vi "FluxMeasure.vi"(4 "On/Off":bool, 5 "error in (no error)":errorcluster, 6 "Gray Image":T1) -> (0 "error out":errorcluster, 1 "实时通量":cluster{"粒子数量":dbl, "粒子数量":dbl, dbl}, 2 "粒子分布":cluster{dbl[], i32[]}, 3 "粒子数量":dbl)   [LabVIEW 2012]
uses:
  <vilib>/vision/Image Controls.llb/IMAQ Image.ctl
  <vilib>/vision/NI_Vision_Development_Module.lvlib
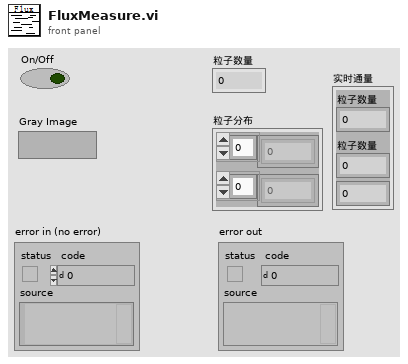
[diagram p1: front panel]
types:
  T1 = typedef "IMAQ Image.ctl" = refnum<image>
  T2 = typedef "Particle Parameters" = i32
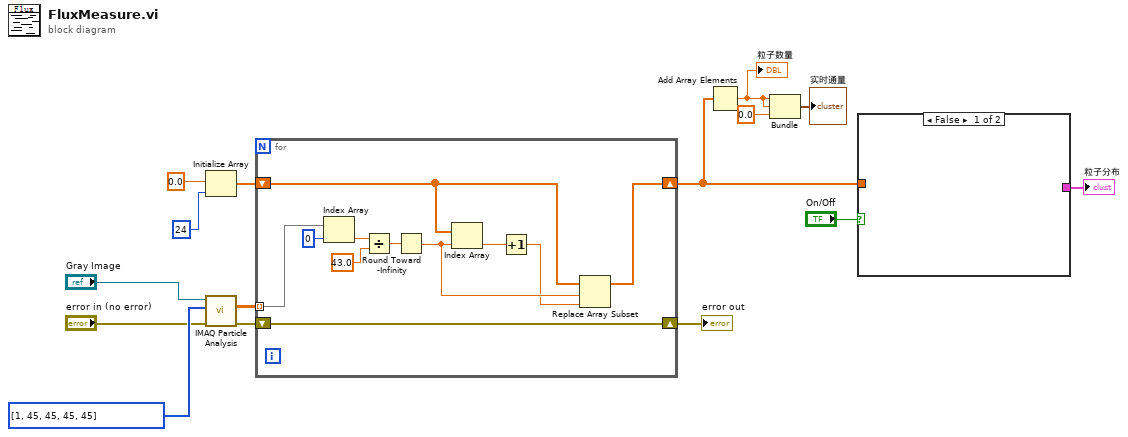
[diagram p0: block diagram]
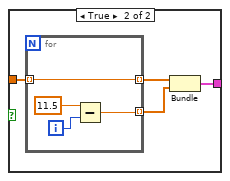
[diagram p2: hidden frame]
diagram:
  w15 = T2[] [1, 45, 45, 45, 45] items=["Center of Mass X", "Center of Mass Y", "First Pixel X", "First Pixel Y", "Bounding Rect Left", "Bounding Rect Top", "Bounding Rect Right", "Bounding Rect Bottom", "Max Feret Diameter Start X", "Max Feret Diameter Start Y", "Max Feret Diameter End X", "Max Feret Diameter End Y", "Max Horiz. Segment Length Left", "Max Horiz. Segment Length Right", "Max Horiz. Segment Length Row", "-", "Bounding Rect Width", "Bounding Rect Height", "Bounding Rect Diagonal", "Perimeter", "Convex Hull Perimeter", "Holes' Perimeter", "Max Feret Diameter", "Equivalent Ellipse Major Axis", "Equivalent Ellipse Minor Axis", "Equivalent Ellipse Minor Axis (Feret)", "Equivalent Rect Long Side", "Equivalent Rect Short Side", "Equivalent Rect Diagonal", "Equivalent Rect Short Side (Feret)", "Average Horiz. Segment Length", "Average Vert. Segment Length", "Hydraulic Radius", "Waddel Disk Diameter", "-", "Area", "Holes' Area", "Particle & Holes' Area", "Convex Hull Area", "Image Area", "-", "Number of Holes", "Number of Horiz. Segments", "Number of Vert. Segments", "-", "Orientation", "Max Feret Diameter Orientation", "-", "% Area/Image Area", "% Area/(Particle & Holes' Area)", "Ratio of Equivalent Ellipse Axes", "Ratio of Equivalent Rect Sides", "-", "Elongation Factor", "Compactness Factor", "Heywood Circularity Factor", "Type Factor", "-", "Sum X", "Sum Y", "Sum XX", "Sum XY", "Sum YY", "Sum XXX", "Sum XXY", "Sum XYY", "Sum YYY", "-", "Moment of Inertia XX", "Moment of Inertia XY", "Moment of Inertia YY", "Moment of Inertia XXX", "Moment of Inertia XXY", "Moment of Inertia XYY", "Moment of Inertia YYY", "Norm. Moment of Inertia XX", "Norm. Moment of Inertia XY", "Norm. Moment of Inertia YY", "Norm. Moment of Inertia XXX", "Norm. Moment of Inertia XXY", "Norm. Moment of Inertia XYY", "Norm. Moment of Inertia YYY", "Hu Moment 1", "Hu Moment 2", "Hu Moment 3", "Hu Moment 4", "Hu Moment 5", "Hu Moment 6", "Hu Moment 7"] ("Pixel Measurements")
  n1 = Initialize Array(0.0 ("粒子数量"), 24 ("维数大小")) -> (w13:dbl[])
  n2 = call "IMAQ Particle Analysis"("error in (no error)"="error in (no error)", "Pixel Measurements"=w15, "Image"="Gray Image") -> ("error out"=w12:errorcluster, "Particle Measurements (Pixels)"=w11:dbl[][])  [unwired: 3 in, 4 out]
  n3 = for {
    tunnel: w11 -> [w22] mode=indexing
    shift-right: [w19] -> w8
    shift-left: w13 -> [w20]
    shift-right: [w18] -> w4
    shift-left: w12 -> [w18]
    n4 = Index Array(array=w22, index=0 ("索引")) -> (element=w25:dbl)
    n5 = Divide(x=w25, y=43.0) -> (x/y=w23:dbl)
    n6 = Round Toward -Infinity(1:w23) -> (0:w21:dbl)
    n7 = Index Array(array=w20, index=w21) -> (element=w17:dbl)
    n8 = Increment(x=w17) -> (x+1=w16:dbl)
    n9 = Replace Array Subset(array=w20, new element=w16, index=w21) -> (w19:dbl[])
  }
  "error out" <- w4
  n10 = Add Array Elements(numeric array=w8) -> (sum=w7:dbl)
  "粒子数量" <- w7
  n11 = Bundle("粒子数量"=w7, "粒子数量"=w7, 0.0) -> (→"实时通量":cluster{"粒子数量":dbl, "粒子数量":dbl, dbl})  [unwired: 1 in]
  n12 = case shown="False" "On/Off" {
    tunnel: [_ w29] -> w10
    tunnel: w8 -> [_ w27]
    frame False {
    }
    frame True {
      n13 = for {
        tunnel: w27 -> [w34] mode=indexing
        tunnel: [w31] -> w30 mode=indexing
        tunnel: [w34] -> w28 mode=indexing
        i -> [w33]
        n14 = Subtract(x=11.5, y=w33) -> (x-y=w31:dbl)
      }
      n15 = Bundle(w28, w30) -> (w29:cluster{dbl[], dbl[]})  [unwired: 1 in]
    }
  }
  "粒子分布" <- w10
